vi "Pos Defender Calc.vi"(0 "Events.Ball out":bool, 1 "IA State Input":T1={"our_robots"=[], "enemy_robots"=[], "balls"=[], "geometry"={"field_length"=0, "field_width"=0, "goal_width"=0, "goal_depth"=0, "center_circle_radius"=0, "defense_width"=0, "defense_depth"=0, "free_kick_from_defense_dist"=0, "penalty_spot_from_field_line_dist"=0, "penalty_line_from_spot_dist"=0, "half_moon_depth"=0, "half_moon_width"=0}, "IA Judge"={"stage"="", "command"="", "our_goalie_id"=0.0, "enemy_goalie_id"=0.0, "command enum"=enum."Halt", "Time"=enum."Azul"}, "Received Timestamp"=timestamp(0 s since 1904-01-01), "Events"={"Touch"=FALSE, "Ball out"=FALSE, "id touch"=0.0, "Ball out of \nVision"=FALSE, "Ball inside \nGoalie area"=FALSE, "Robot not responding"=FALSE, "Robots responding status"=[1.0, 1.0, 1.0, 1.0, 1.0, 1.0], "Enemy Ball \nPossession"=FALSE, "Pass State"=FALSE, "id end of pass"=0.0, "Kick"=FALSE, "Id ini Possession"=0.0, "Ball Possesion"=FALSE, "Id Possesion"=0.0}}, 4 "AI Parameters":T12={"GotoKick"={"Dist do cone a frente"=150.0, "attacker farback"=1500.0, "Perto"=300.0, "min dist to kick"=150.0, "kick eps"=0.0, "Time to transition"=0.05}, "Attacker"={"CC chute"=0.09, "CC passe"=0.045, "Kick Force"=100.0, "D ball-robot Kick"=200.0, "D ball-robot Pass"=0.3}, "Defender"={"D max"=1700.0, "Vel p/ robô av"=1000.0, "Kick Force"=100.0, "D atk-def"=0.0, "D farback"=0.0}, "Timeout"={"Field/v in x"=6.0, "Dist Robots"=300, "Dist up in y"=300}, "Pose Striker"={"dist"=200.0, "Numeric"=-4.0, "dist 2"=200.0}, "Dist Stop"=300.0, "Distance when ball out"=200, "D central gap "=150.0, "T pass"=0.0, "Force ++"=0.0, "range kick"=0.0, "Chute alto"=TRUE, "Marcador novo"=TRUE} {"D central gap" format="%#_13g"; "Dist Stop" format="%#_13g"; "Pose Striker"."Numeric" format="%#_13g"; "Defender"."Kick Force" format="%#_13g"; "Defender"."Vel p/ robô av" format="%#_13g"; "Attacker"."D ball-robot Kick" format="%#_13g"; "Attacker"."Kick Force" format="%#_13g"; "Attacker"."CC passe" format="%#_13g"; "Attacker"."CC chute" format="%#_13g"; "GotoKick"."kick eps" format="%#_13g"; "GotoKick"."min dist to kick" format="%#_13g"; "GotoKick"."Perto" format="%#_13g"; "GotoKick"."attacker farback" format="%#_13g"; "GotoKick"."Dist do cone a frente" format="%#_13g"}, 5 "Stop?":bool, 6 "Field defense":dbl[](array[numeric]), 7 "Real Ball":dbl[](array[numeric]), 8 "Field Size in":T13, 9 "Defensores":u32[](array[numeric]), 10 "Ball":dbl[](array[numeric]), 11 "total":i32) -> (2 "Posição dos Defensores":dbl[][](array[numeric]), 3 "Central Position":dbl[](array[numeric]))   [LabVIEW 2017]
uses:
  Core/Field Size.ctl
  AI Parameters.ctl
  Functions Enum.ctl
  AttackerStates.ctl
  Core/AI Robot.ctl
  Core/AI Ball.ctl
  Command Enum.ctl
  Core/AI Judge.ctl
  Util/Events/Events.ctl
  Core/AI Input.ctl
  Path Planning/RRT/PathDest.ctl
  Path Planning/RRT/PathDests.ctl
panel:
  in  "Array 2":dbl[][](array[numeric])=[[99999.0, 99999.0], [99999.0, 99999.0], [99999.0, 99999.0], [99999.0, 99999.0], [99999.0, 99999.0], [99999.0, 99999.0], [99999.0, 99999.0]]
  in  "Array":dbl[][](array[numeric])=[[99999.0, 99999.0], [99999.0, 99999.0], [99999.0, 99999.0], [99999.0, 99999.0], [99999.0, 99999.0], [99999.0, 99999.0], [99999.0, 99999.0]]
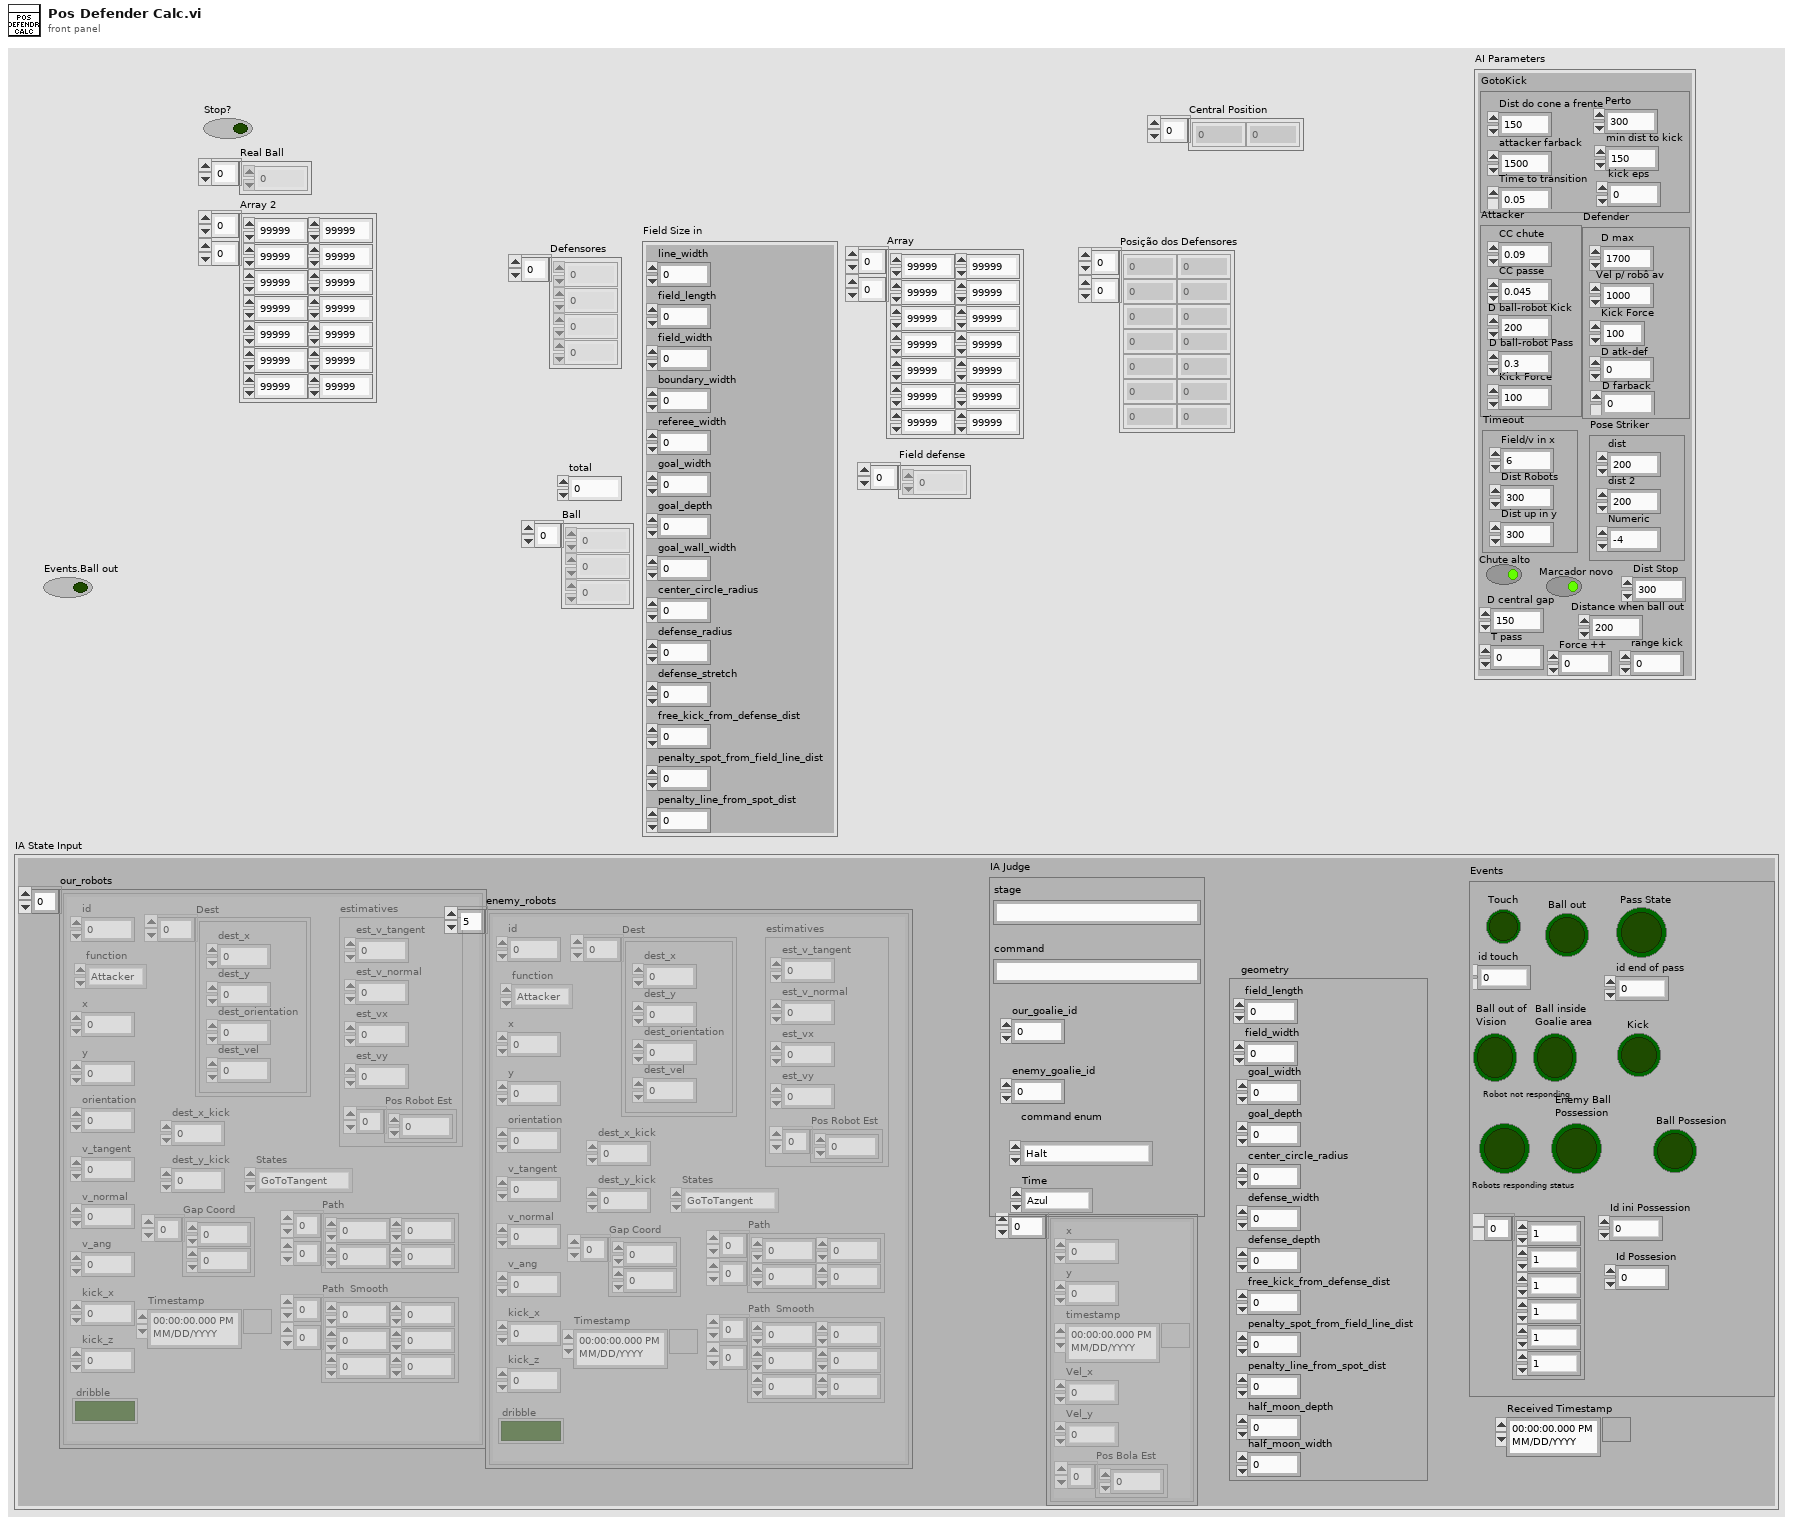
[diagram p1: front panel]
types:
  T1 = typedef "AI Input.ctl" = cluster{"our_robots":T2[], "enemy_robots":T2[], "balls":T7[], "geometry":T8, "IA Judge":T9, "Received Timestamp":timestamp, "Events":T11}
  T2 = typedef "AI Robot.ctl" = cluster{"id":u32, "function":T3, "x":dbl, "y":dbl, "orientation":dbl, "v_tangent":dbl, "v_normal":dbl, "v_ang":dbl, "kick_x":dbl, "kick_z":dbl, "dribble":bool, "Timestamp":timestamp, "estimatives":cluster{"est_v_tangent":dbl, "est_v_normal":dbl, "est_vx":dbl, "est_vy":dbl, "Pos Robot Est":dbl[]}, "dest_x_kick":dbl, "dest_y_kick":dbl, "Gap Coord":dbl[], "States":T4, "Path ":dbl[][], "Path  Smooth":dbl[][], "Dest":T5}
  T3 = typedef "Functions Enum.ctl" = enum16{"Attacker", "Goalie", "Defender", "Striker", "Goto 0", "Dummy", "Kicker", "ZigZag"}
  T4 = typedef "AttackerStates.ctl" = enum16{"Pass", "GoToTangent", "BallGetting", "GoToKick", ""}
  T5 = typedef "PathDests.ctl" = T6[]
  T6 = typedef "PathDest.ctl" = cluster{"dest_x":dbl, "dest_y":dbl, "dest_orientation":dbl, "dest_vel":dbl}
  T7 = typedef "AI Ball.ctl" = cluster{"x":dbl, "y":dbl, "timestamp":timestamp, "Vel_x":dbl, "Vel_y":dbl, "Pos Bola Est":dbl[]}
  T8 = typedef "Field Size.ctl" = cluster{"field_length":u32, "field_width":u32, "goal_width":u32, "goal_depth":u32, "center_circle_radius":u32, "defense_width":u32, "defense_depth":u32, "free_kick_from_defense_dist":u32, "penalty_spot_from_field_line_dist":u32, "penalty_line_from_spot_dist":u32, "half_moon_depth":u32, "half_moon_width":u32}
  T9 = typedef "AI Judge.ctl" = cluster{"stage":string, "command":string, "our_goalie_id":dbl, "enemy_goalie_id":dbl, "command enum":T10, "Time":enum16{"Azul", "Amarelo"}}
  T10 = typedef "Command Enum.ctl" = enum16{"Halt", "Stop", "Force Start", "PKA Normal Start", "Prepare Kickoff Ally", "PKE Normal Start", "Prepare Kickoff Enemy", "Prepare Penalty Ally", "PPA Normal Start", "Prepare Penalty Enemy", "PPE Normal Start", "Direct Free Enemy", "Direct Free Ally", "Indirect Free Enemy", "Indirect Free Ally", "Timeout Enemy", "Timeout Ally", "Goal Enemy", "Goal Ally", "Ball Placement Enemy", "Ball Placement Ally", "Normal Half Time", "Extra Time Break", "Extra Half Time", "None", "Post Game"}
  T11 = typedef "Events.ctl" = cluster{"Touch":bool, "Ball out":bool, "id touch":dbl, "Ball out of \nVision":bool, "Ball inside \nGoalie area":bool, "Robot not responding":bool, "Robots responding status":dbl[], "Enemy Ball \nPossession":bool, "Pass State":bool, "id end of pass":dbl, "Kick":bool, "Id ini Possession":dbl, "Ball Possesion":bool, "Id Possesion":dbl}
  T12 = typedef "AI Parameters.ctl" = cluster{"GotoKick":cluster{"Dist do cone a frente":dbl, "attacker farback":dbl, "Perto":dbl, "min dist to kick":dbl, "kick eps":dbl, "Time to transition":dbl}, "Attacker":cluster{"CC chute":dbl, "CC passe":dbl, "Kick Force":dbl, "D ball-robot Kick":dbl, "D ball-robot Pass":dbl}, "Defender":cluster{"D max":dbl, "Vel p/ robô av":dbl, "Kick Force":dbl, "D atk-def":dbl, "D farback":dbl}, "Timeout":cluster{"Field/v in x":dbl, "Dist Robots":u32, "Dist up in y":u32}, "Pose Striker":cluster{"dist":dbl, "Numeric":dbl, "dist 2":dbl}, "Dist Stop":dbl, "Distance when ball out":i32, "D central gap ":dbl, "T pass":dbl, "Force ++":dbl, "range kick":dbl, "Chute alto":bool, "Marcador novo":bool}
  T13 = typedef "Field Size.ctl" = cluster{"line_width":u32, "field_length":u32, "field_width":u32, "boundary_width":u32, "referee_width":u32, "goal_width":u32, "goal_depth":u32, "goal_wall_width":u32, "center_circle_radius":u32, "defense_radius":u32, "defense_stretch":u32, "free_kick_from_defense_dist":u32, "penalty_spot_from_field_line_dist":u32, "penalty_line_from_spot_dist":u32}
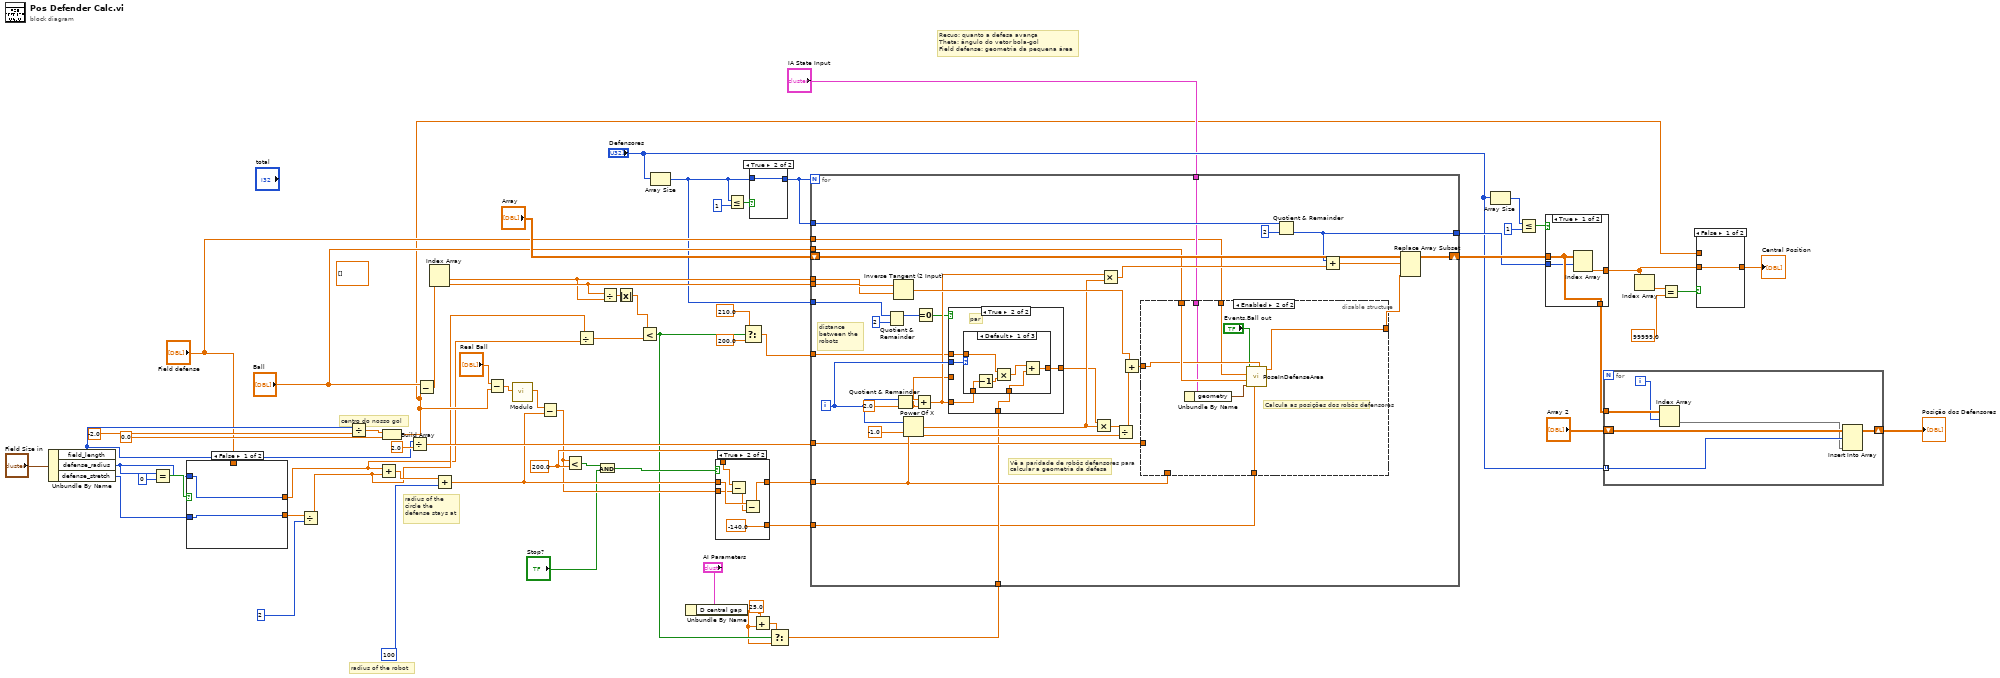
[diagram p0: block diagram]
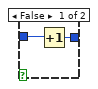
[diagram p2: hidden frame]
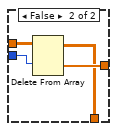
[diagram p3: hidden frame]
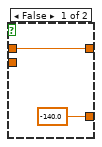
[diagram p5: hidden frame]
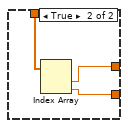
[diagram p6: hidden frame]
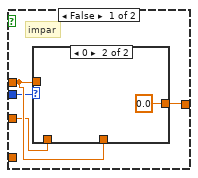
[diagram p7: hidden frame]
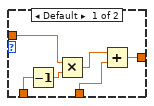
[diagram p8: hidden frame]
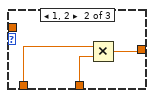
[diagram p9: hidden frame]
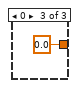
[diagram p10: hidden frame]
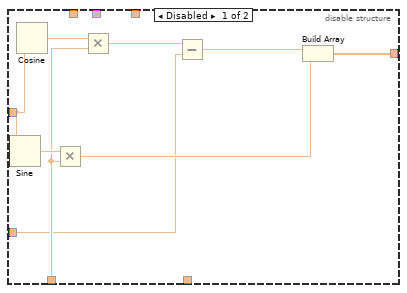
[diagram p11: hidden frame]
diagram:
  (unwired) dbl[][] [] ("Array")
  w47 = 200.0 ("y")
  # "Recuo: quanto a defesa avança\nTheta: ângulo do vetor bola-gol\nField defense: geometria da pequena área"
  # "radius of the circle the defense stays at"
  # "centro do nosso gol"
  # "radius of the robot"
  n1 = Unbundle By Name("Field Size in") -> ("field_length"=w58:u32, "defense_radius"=w54:u32, "defense_stretch"=w53:u32)
  n2 = Equal?(x=w54, y=u32 0) -> (x = y?=w55:bool)
  n3 = case shown="False" w55 {
    tunnel: [w68 w71] -> w16
    tunnel: w54 -> [w68 _]
    tunnel: w53 -> [w67 _]
    tunnel: [w67 w70] -> w52
    tunnel: "Field defense" -> [_ w69]
    frame False {
    }
    frame True {
      n4 = Index Array(array=w69) -> (element #1=w71:dbl, element #2=w70:dbl)  [unwired: 2 in]
    }
  }
  n5 = Divide(x=w52, y=u32 2) -> (x/y=w17:dbl)
  n6 = Divide(x=w58, y=-2.0) -> (x/y=w63:dbl)
  n7 = Add(x=w16, y=w17) -> (x+y=w65:dbl)
  n8 = Build Array(w63, 0.0 ("element")) -> (w18:dbl[])
  n9 = Divide(x=w58, y=2.0) -> (x/y=w57:dbl)
  n10 = Subtract(x="Ball", y=w18) -> (x-y=w51:dbl[])
  n11 = Index Array(array=w51) -> (element #1=w14:dbl, element #2=w15:dbl)  [unwired: 2 in]
  n12 = Add(x=w65, y=u32 100) -> (x+y=w49:dbl)
  n13 = Subtract(x="Real Ball", y=w18) -> (x-y=w42:dbl[])
  n14 = call "Modulo.vi"("2D vector"=w42) -> ("Modulo"=w50:dbl)  [unwired: 10 in]
  n15 = Subtract(x=w50, y=w49) -> (x-y=w46:dbl)
  n16 = Less?(x=w46, y=w47) -> (x < y?=w45:bool)
  n17 = Divide(x=w17, y=w16) -> (x/y=w11:dbl)
  n18 = And(x=w45, y="Stop?") -> (x .and. y?=w44:bool)
  n19 = Divide(x=w15, y=w14) -> (x/y=w13:dbl)
  n20 = Absolute Value(x=w13) -> (abs(x)=w12:dbl)
  n21 = Less?(x=w12, y=w11) -> (x < y?=w7:bool)
  n22 = Array Size(array="Defensores") -> (size(s)=w1:i32)
  n23 = Unbundle By Name("AI Parameters") -> ("D central gap"=w4:dbl)
  n24 = case shown="True" w44 {
    tunnel: w49 -> [w73 w79]
    tunnel: [w73 w76] -> w48
    tunnel: w47 -> [_ w78]
    tunnel: w46 -> [_ w77]
    tunnel: [-140.0 -140.0] -> w20
    frame False {
    }
    frame True {
      n25 = Subtract(x=w78, y=w77) -> (x-y=w75:dbl)
      n26 = Subtract(x=w79, y=w75) -> (x-y=w76:dbl)
    }
  }
  n27 = Less Or Equal?(x=w1, y=1) -> (x <= y?=w23:bool)
  n28 = Select(t=210.0, s=w7, f=200.0) -> (s? t:f=w8:dbl)
  n29 = case shown="True" w23 {
    tunnel: w1 -> [w81 w82]
    tunnel: [w80 w82] -> w29
    frame False {
      n30 = Increment(x=w81) -> (x+1=w80:i32)
    }
    frame True {
    }
  }
  n31 = Add(x=25.0, y=w4) -> (x+y=w2:dbl)
  n32 = Select(t=w2, s=w7, f=w4) -> (s? t:f=w6:dbl)
  n33 = for {
    N: w29 -> [_]
    tunnel: w15 -> [w116]
    tunnel: w14 -> [w115]
    tunnel: w48 -> [w109]
    shift-right: [w104] -> w32
    shift-left: "Array" -> [w103]
    tunnel: w57 -> [w108]
    tunnel: [w98] -> w31
    tunnel: w29 -> [w97]
    tunnel: w6 -> [w93]
    tunnel: "Ball" -> [w92]
    tunnel: "IA State Input" -> [w91]
    tunnel: "Field defense" -> [w90]
    tunnel: w20 -> [w89]
    tunnel: w8 -> [w88]
    tunnel: w1 -> [w87]
    i -> [w96]
    # "Vê a paridade de robôs defensores para\ncalcular a geometria da defesa"
    # "distance between the robots"
    n34 = Quotient & Remainder(x=w87, y=2) -> (x-y*floor(x/y)=w85:i32)  [unwired: 1 out]
    n35 = Inverse Tangent (2 Input)(1:w115, 2:w116) -> (0:w112:dbl)
    n36 = Quotient & Remainder(x=w96, y=2.0) -> (x-y*floor(x/y)=w106:dbl, floor(x/y)=w83:dbl)
    n37 = Power Of X(1:-1.0, 2:w96) -> (0:w102:dbl)
    n38 = Add(x=w106, y=w83) -> (x+y=w95:dbl)
    n39 = Equal To 0?(x=w85) -> (x = 0?=w84:bool)
    n40 = case shown="True" w84 {
      tunnel: w96 -> [w118 w132]
      tunnel: w95 -> [_ w131]
      tunnel: [w119 w130] -> w94
      tunnel: w93 -> [_ w129]
      tunnel: w88 -> [w120 w128]
      tunnel: w83 -> [w117 _]
      frame False {
        # "impar"
        n41 = case shown="0" w118 {
          tunnel: [w124 0.0 ("x")] -> w119
          tunnel: w117 -> [w126 _]
          tunnel: w120 -> [w122 _]
          tunnel: w120 -> [w121 _]
          frame Default {
            n42 = Decrement(x=w126) -> (x-1=w125:dbl)
            n43 = Multiply(x=w121, y=w125) -> (x*y=w123:dbl)
            n44 = Add(x=w123, y=w122) -> (x+y=w124:dbl)
          }
          frame 0 {
          }
        }
      }
      frame True {
        # "par"
        n45 = case shown="Default" w132 {
          tunnel: [w136 w139 0.0 ("x")] -> w130
          tunnel: w131 -> [w138 w141 _]
          tunnel: w129 -> [w134 w140 _]
          tunnel: w128 -> [w133 _ _]
          frame Default {
            n46 = Decrement(x=w138) -> (x-1=w137:dbl)
            n47 = Multiply(x=w133, y=w137) -> (x*y=w135:dbl)
            n48 = Add(x=w135, y=w134) -> (x+y=w136:dbl)
          }
          frame 1, 2 {
            n49 = Multiply(x=w141, y=w140) -> (x*y=w139:dbl)
          }
          frame 0 {
          }
        }
      }
    }
    n50 = Multiply(x=w94, y=w102) -> (x*y=w113:dbl)
    n51 = Multiply(x=w95, y=w102) -> (x*y=w100:dbl)
    n52 = Divide(x=w113, y=w109) -> (x/y=w111:dbl)
    n53 = Add(x=w112, y=w111) -> (x+y=w110:dbl)
    n54 = disable-structure shown="Enabled" {
      disable-tunnel: w110 -> [w151 w158]
      disable-tunnel: w109 -> [w147 _]
      disable-tunnel: w108 -> [w144 _]
      disable-tunnel: [w143 w157] -> w105
      disable-tunnel: w92 -> [_ w159]
      disable-tunnel: w91 -> [_ w154]
      disable-tunnel: w90 -> [_ w155]
      disable-tunnel: w89 -> [_ w152]
      frame Disabled {
        n55 = Sine(x=w151) -> (sin(x)=w149:dbl)
        n56 = Cosine(x=w151) -> (cos(x)=w150:dbl)
        n57 = Multiply(x=w149, y=w147) -> (x*y=w145:dbl)
        n58 = Multiply(x=w150, y=w147) -> (x*y=w148:dbl)
        n59 = Subtract(x=w148, y=w144) -> (x-y=w146:dbl)
        n60 = Build Array(w146, w145) -> (w143:dbl[])
      }
      frame Enabled {
        # "Calcula as posições dos robôs defensores"
        n61 = Unbundle By Name(w154) -> ("geometry"=w156:T8)
        n62 = call "PoseInDefenseArea.vi"("theta"=w158, "Recuo"=w152, "geometry"=w156, "Ball"=w159, "Field defense"=w155, "Events.Ball out"="Events.Ball out") -> ("Array"=w157:dbl[])  [unwired: 5 in]
      }
    }
    n63 = Quotient & Remainder(x=w97, y=2) -> (floor(x/y)=w98:i32)  [unwired: 1 out]
    n64 = Add(x=w98, y=w100) -> (x+y=w101:dbl)
    n65 = Replace Array Subset(array=w103, new element=w105, index (row)=w101) -> (w104:dbl[][])  [unwired: 1 in]
  }
  n66 = Array Size(array="Defensores") -> (size(s)=w26:i32)
  n67 = Less Or Equal?(x=w26, y=1) -> (x <= y?=w27:bool)
  n68 = case shown="True" w27 {
    tunnel: [w162 w166] -> w34
    tunnel: w32 -> [w161 w165]
    tunnel: w31 -> [w160 w164]
    tunnel: [w161 w163] -> w30
    frame True {
      n69 = Index Array(array=w161, index (row)=w160) -> (element=w162:dbl[])  [unwired: 1 in]
    }
    frame False {
      n70 = Delete From Array(array=w165, index (row)=w164) -> (deleted portion=w166:dbl[], array with subset deleted=w163:dbl[][])  [unwired: 2 in]
    }
  }
  n71 = for {
    tunnel: "Defensores" -> [w171] mode=indexing
    shift-right: [w170] -> w39
    shift-left: "Array 2" -> [w172]
    tunnel: w30 -> [w169]
    i -> [w168]
    n72 = Index Array(array=w169, index (row)=w168) -> (element=w167:dbl[])  [unwired: 1 in]
    n73 = Insert Into Array(array=w172, index (row)=w171, new element=w167) -> (w170:dbl[][])  [unwired: 1 in]
  }
  "Posição dos Defensores" <- w39
  n74 = Index Array(array=w34) -> (element=w36:dbl)  [unwired: 1 in]
  n75 = Equal?(x=w36, y=99999.0) -> (x = y?=w33:bool)
  n76 = case shown="False" w33 {
    tunnel: [w173 w174] -> w37
    tunnel: w34 -> [w173 _]
    tunnel: w18 -> [_ w174]
    frame False {
    }
    frame True {
    }
  }
  "Central Position" <- w37
